vi "Untitled 1.vi"() -> ()   [LabVIEW 2021]
panel:
  out "answer":bool
  in  "x4":bool
  out "information":string
  in  "x3":bool
  in  "x2":bool
  in  "x1":bool
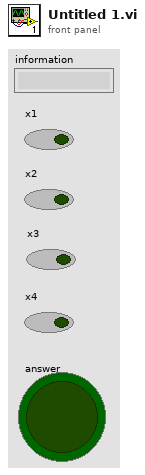
[diagram p1: front panel]
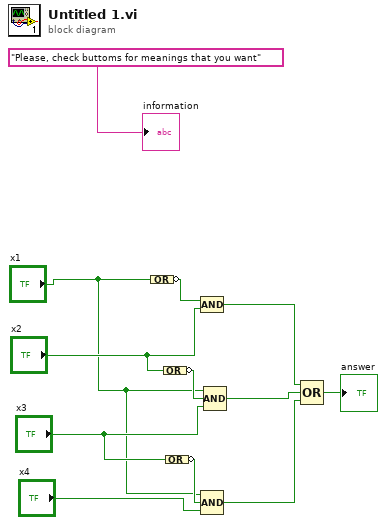
[diagram p0: block diagram]
diagram:
  n1 = Compound Arithmetic op=OR("x1") -> (invert w11:bool)
  n2 = Compound Arithmetic op=OR("x2") -> (invert w9:bool)
  n3 = Compound Arithmetic op=OR("x3") -> (invert w7:bool)
  n4 = Compound Arithmetic op=AND(w11, "x2") -> (w4:bool)
  n5 = Compound Arithmetic op=AND("x1", w7, "x4") -> (w2:bool)
  n6 = Compound Arithmetic op=AND("x1", w9, "x3") -> (w3:bool)
  n7 = Compound Arithmetic op=OR(w4, w3, w2) -> (→"answer":bool)
  "information" <- "Please, check buttoms for meanings that you want"
